vi "Digital Bank Write.vi"(6 "timeout ms (10)":i32=10, 8 "error in (no error)":errorcluster, 9 "Channels to set":i32[](array[numeric]), 10 "Value to set":bool, 11 "TCP Network Connection in":refnum<k5>) -> (0 "error out":errorcluster, 3 "TCP Network Connection out":refnum<k5>)   [LabVIEW 2024, in "OptoMMP.lvlib"]
doc: "Performs a digital bank read on the specified TCP network. Writes the provided boolean value to the specified channels. \n\n\"Channels to set\" corresponds to points 0-63, for a total of 64 channels. Each module begins on the order of 4 points (module 0 starts at point 0, module 1 starts at point 4, etc.). \"Digital Bank Write\" must be preceded by \"OptoMMP Open Connection\".\n\nLast updated: 8/6/2025"
uses:
  <instrlib>/OptoMMP/OptoMMP.lvlib
panel:
  # "Copyright (c) 2025 California Institute of Technology (Caltech).\nU.S. Government sponsorship acknowledged.\n\nLicensed under the Apache License, Version 2.0 (the \"License\");\nyou may not use this file except in compliance with the License.\nYou may obtain a copy of the License at\n\n    http://www.apache.org/licenses/LICENSE-2.0\n\nUnless required by applicable law or agreed to in writing, software\ndistributed under the License is distributed on an \"AS IS\" BASIS,\nWITHOUT WARRANTIES OR CONDITIONS OF ANY KIND, either express or implied.\nSee the License for the specific language governing permissions and\nlimitations under the License."
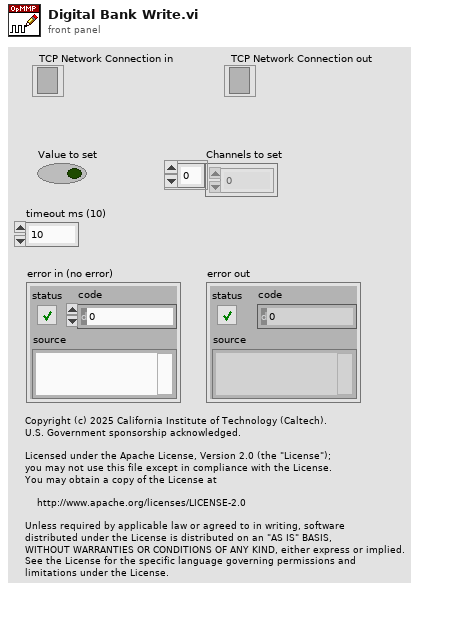
[diagram p1: front panel]
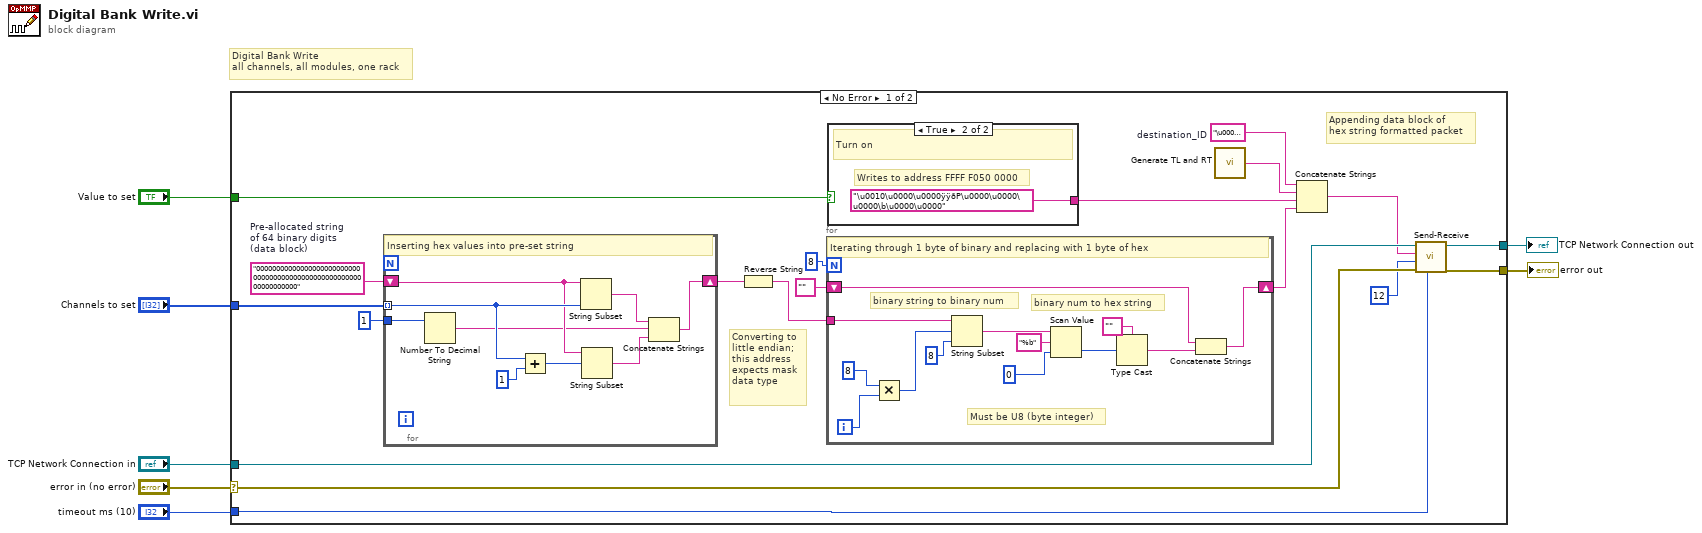
[diagram p0: block diagram]
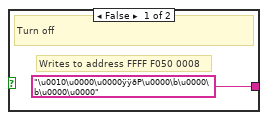
[diagram p2: hidden frame]
diagram:
  # "Digital Bank Write\nall channels, all modules, one rack"
  n1 = case shown="No Error" "error in (no error)" {
    selector: "error in (no error)" -> [w13 w51]
    tunnel: "Channels to set" -> [w26 _]
    tunnel: "Value to set" -> [w20 _]
    tunnel: [w9 w51] -> w5
    tunnel: [w10 w52] -> w4
    tunnel: "TCP Network Connection in" -> [w14 w52]
    tunnel: "timeout ms (10)" -> [w8 _]
    frame No Error {
      w16 = "\u0000\u0000"  # destination_ID
      w17 = "0000000000000000000000000000000000000000000000000000000000000000"  # Pre-allocated string  of 64 binary digits (data block)
      # "Converting to\nlittle endian;\nthis address \nexpects mask\ndata type"
      # "Appending data block of\nhex string formatted packet"
      n2 = for {
        tunnel: w26 -> [w33] mode=indexing
        tunnel: i16 1 -> [w31]
        shift-right: [w29] -> w25
        shift-left: w17 -> [w32]
        # "Inserting hex values into pre-set string"
        n3 = Number To Decimal String(number=w31) -> (decimal integer string=w30:string)  [unwired: 1 in]
        n4 = Add(x=w33, y=1) -> (x+y=w36:i32)
        n5 = String Subset(string=w32, length (rest)=w33) -> (substring=w35:string)  [unwired: 1 in]
        n6 = String Subset(string=w32, offset (0)=w36) -> (substring=w34:string)  [unwired: 1 in]
        n7 = Concatenate Strings(w35, w30, w34) -> (w29:string)
      }
      n8 = Reverse String(1:w25) -> (0:w24:string)
      n9 = for {
        N: 8 -> [_]
        tunnel: w24 -> [w46]
        shift-right: [w39] -> w22
        shift-left: "" -> [w38]
        i -> [w49]
        # "Must be U8 (byte integer)"
        # "binary num to hex string"
        # "binary string to binary num"
        # "Iterating through 1 byte of binary and replacing with 1 byte of hex"
        n10 = Multiply(x=8, y=w49) -> (x*y=w47:i32)
        n11 = String Subset(string=w46, offset (0)=w47, length (rest)=8 ("length (rest)")) -> (substring=w42:string)
        n12 = Scan Value(string=w42, format string="%b", default (0 dbl)=u8 0) -> (value=w43:u8)  [unwired: 1 out]
        n13 = Type Cast(type="", x=w43) -> (*(type *) &x=w40:string)
        n14 = Concatenate Strings(w38, w40) -> (w39:string)
      }
      n15 = case shown="True" w20 {
        tunnel: ["\u0010\u0000\u0000ÿÿðP\u0000\b\u0000\b\u0000\u0000" "\u0010\u0000\u0000ÿÿðP\u0000\u0000\u0000\b\u0000\u0000"] -> w19
        frame False {
          # "Writes to address FFFF F050 0008"
          # "Turn off"
        }
        frame True {
          # "Writes to address FFFF F050 0000"
          # "Turn on"
        }
      }
      n16 = call <instrlib>:"Generate TL and RT.vi"() -> ("tl + rt"=w15:string)
      n17 = Concatenate Strings(w16, w15, w19, w22) -> (w11:string)
      n18 = call <instrlib>:"Send-Receive.vi"("timeout ms (10)"=w8, "error in (no error)"=w13, "bytes to read"=12, "request packet"=w11, "TCP Network Connection in"=w14) -> ("error out"=w9:errorcluster, "connection ID out"=w10:refnum<k5>)  [unwired: 4 in, 1 out]
    }
    frame Error {
    }
  }
  "error out" <- w5
  "TCP Network Connection out" <- w4
